vi "Determine Correct Order.vi"(10 "Right Side":T1[](array[typedef]), 11 "Left Side":T1[](array[typedef])) -> (3 "Correct Order":bool)   [LabVIEW 2020]
uses:
  ENUM_Item Type.ctl
  Control 2.ctl
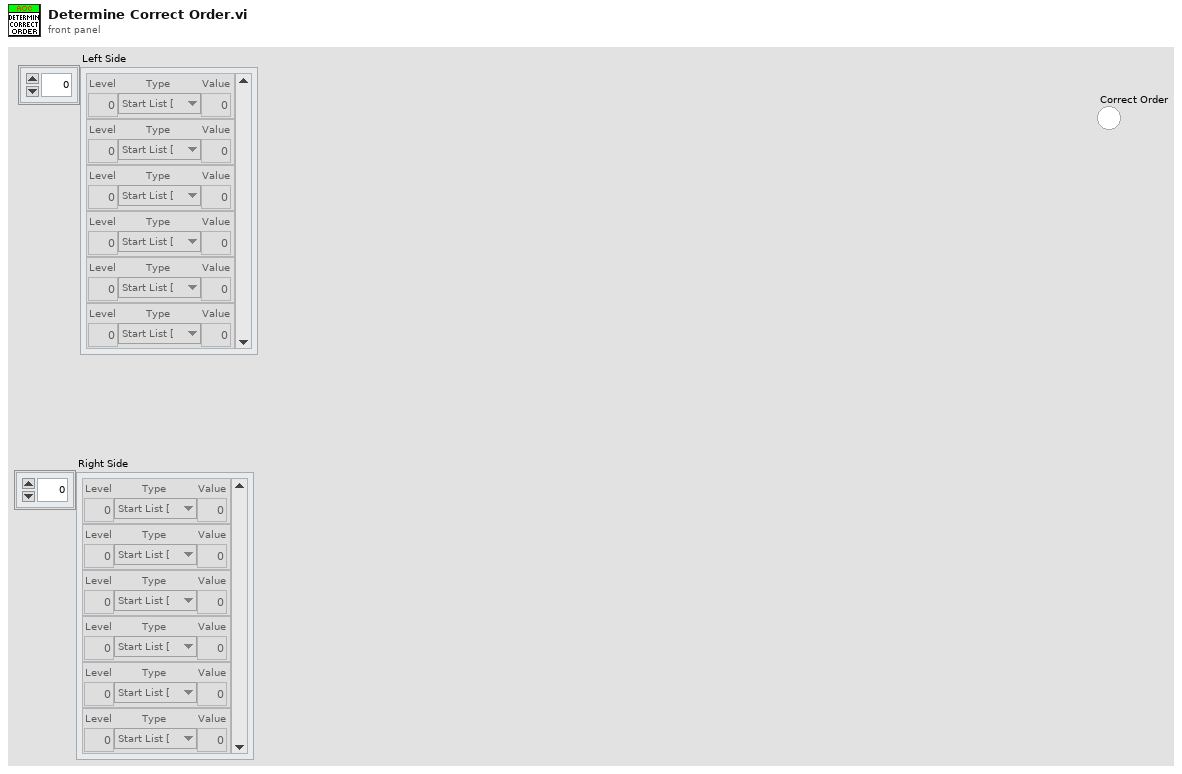
[diagram p1: front panel]
types:
  T1 = typedef "Control 2.ctl" = cluster{"Level":i32, "Type":T2, "Value":i32}
  T2 = typedef "ENUM_Item Type.ctl" = enum16{"Start List [", "Integer", "End List ]"}
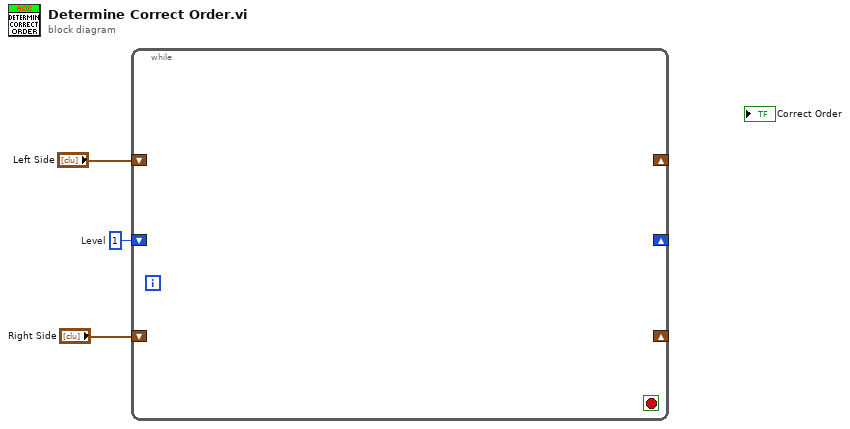
[diagram p0: block diagram]
diagram:
  w1 = 1  # Level
  n1 = while {
    shift-right: _ -> [_]
    shift-left: w1 -> [_]
    shift-right: _ -> [_]
    shift-left: "Left Side" -> [_]
    shift-right: _ -> [_]
    shift-left: "Right Side" -> [_]
    stop <- _ stop-if-true
  }
